vi "Main.vi"() -> ()   [LabVIEW 2019, in "Configuration.lvlib"]
uses:
  Configuration.lvlib
  Typedefs/Module References.ctl
  Typedefs/Enum_Module_Name.ctl
  Typedefs/Message.ctl
  Typedefs/Main Configuration States.ctl
  Typedefs/Configuration.ctl
  Typedefs/Application Configuration.ctl
  Module Template/Typedefs/Config.ctl
  Module Template/SubVIs/Module Template Configuraton Extractor API.vi
  Architecture.lvlib
  Module Template/Module Template.lvlib
panel:
  in  "Module_Refs":T1={"ModuleName"=enum."Controller", "Queue"=refnum, "user event"=refnum, "VI Refnum"=refnum, "ShowFP"=FALSE, "StatesTracking Enabled"=FALSE}
  out "error out":errorcluster
  in  "error in (no error)":errorcluster
  out "Message":string
  in  "Stop App":bool
  in  "Stop Module":bool
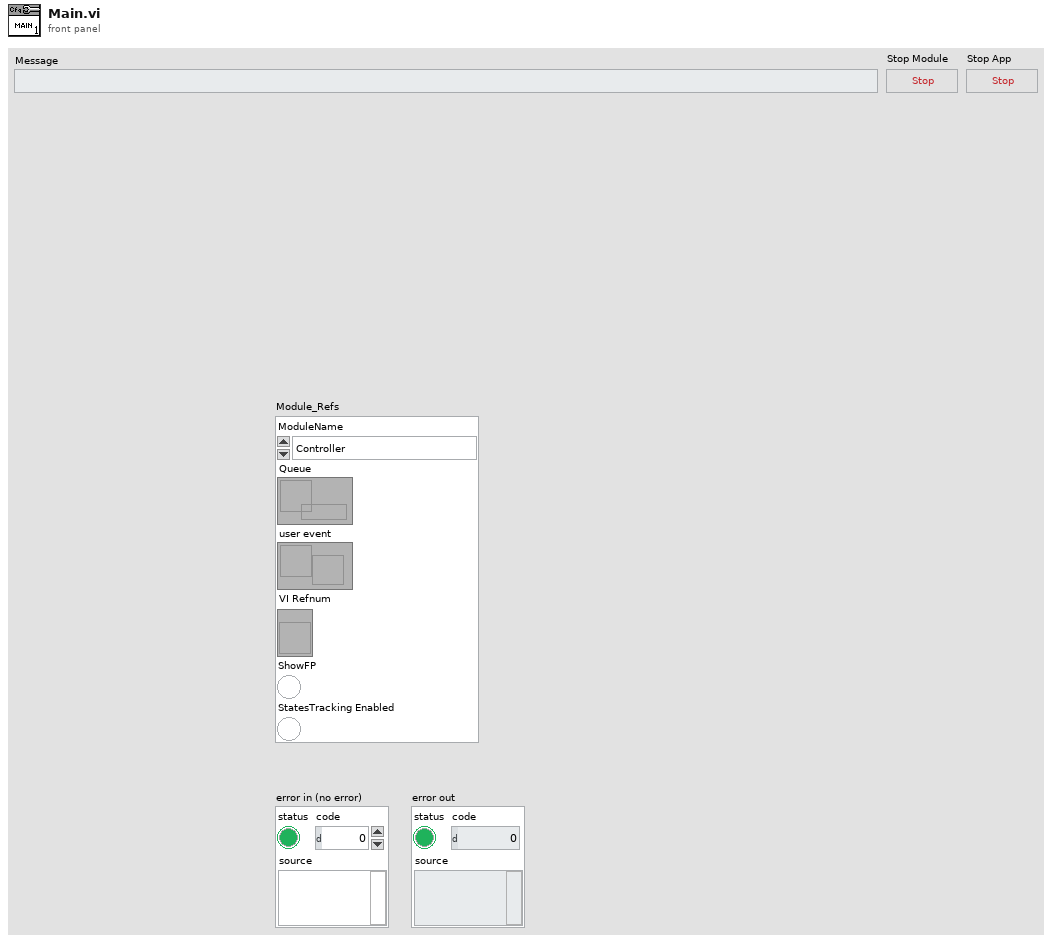
[diagram p1: front panel]
types:
  T1 = typedef "Architecture.lvlib/Module References.ctl" = cluster{"ModuleName":T2, "Queue":refnum<queue>, "user event":refnum<user-event>, "VI Refnum":refnum<vi>, "ShowFP":bool, "StatesTracking Enabled":bool}
  T2 = typedef "Architecture.lvlib/Enum_Module_Name.ctl" = enum16{"Configuration", "Error_Handler", "Log", "Database", "Controller", "User Console", "Display Console", "Sensor Interface"}
  T3 = typedef "Configuration.lvlib/Main Configuration States.ctl" = cluster{"Module_Refs":T1, "Response Data":variant, "Configuration":T4}
  T4 = typedef "Configuration.lvlib/Configuration.ctl" = cluster{"Enabled":bool}
  T5 = enum32{"Invalid", "Standard", "Closed", "Hidden", "Minimized", "Maximized"}
  T6 = typedef "Architecture.lvlib/Module Template.lvlib/Config.ctl" = cluster{"Module Enabled":bool}
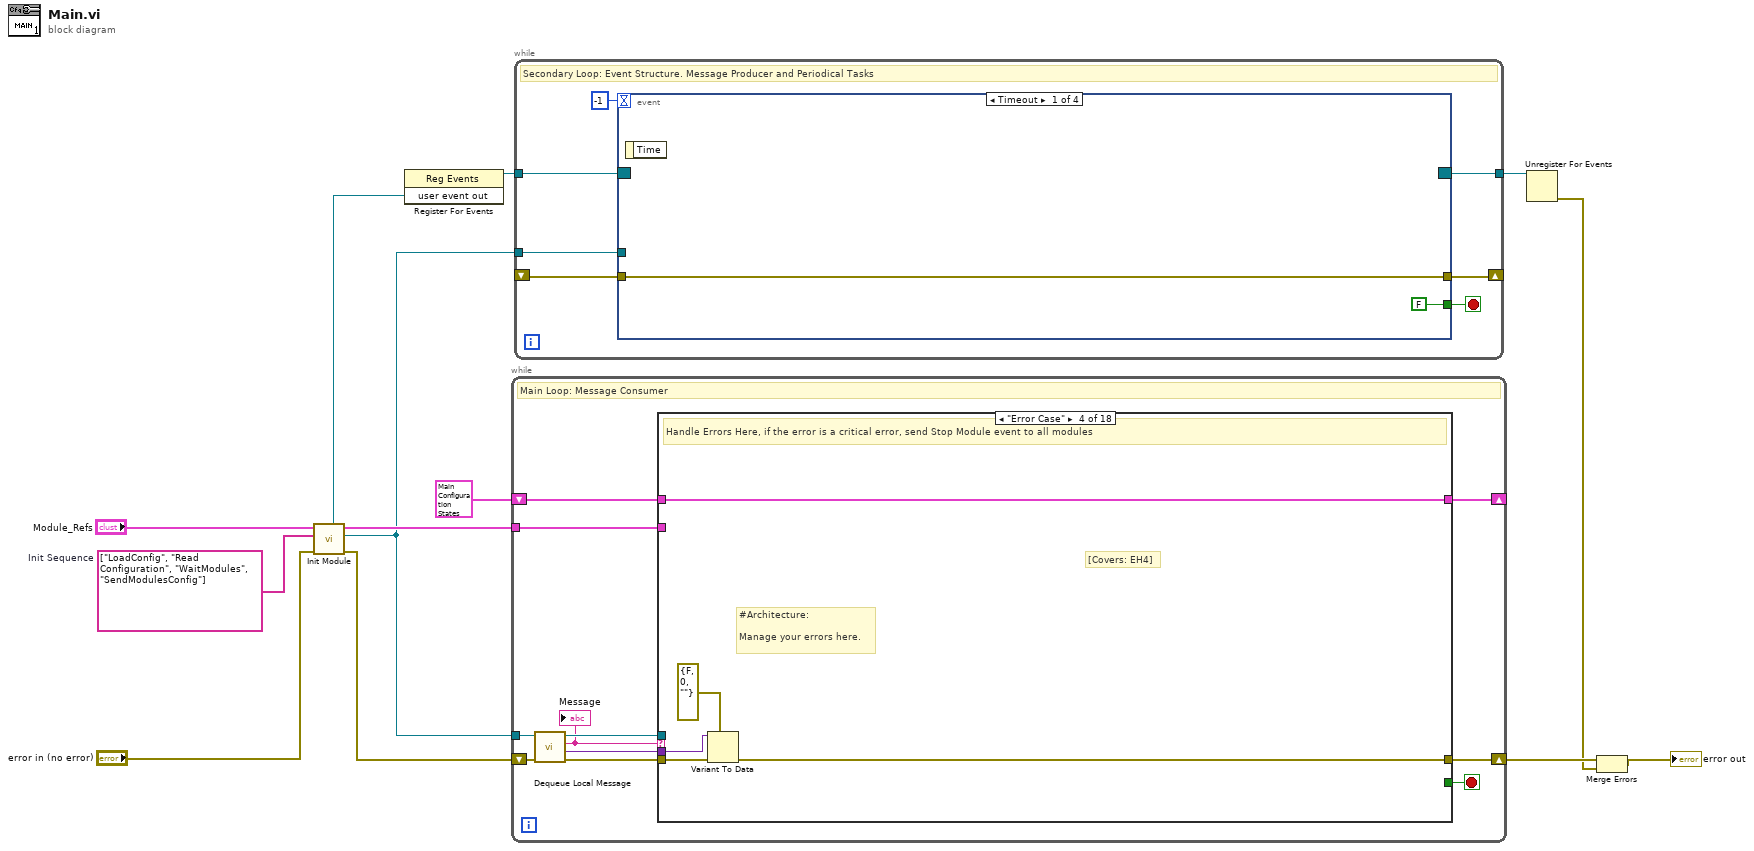
[diagram p0: block diagram]
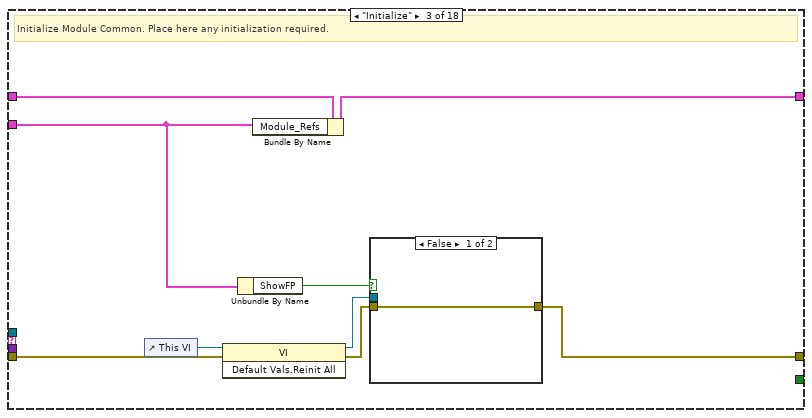
[diagram p4: hidden frame]
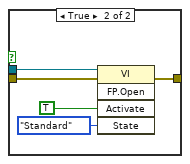
[diagram p5: hidden frame]
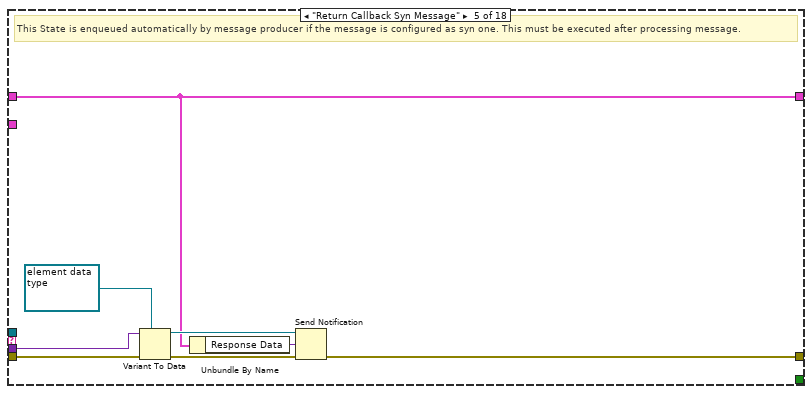
[diagram p6: hidden frame]
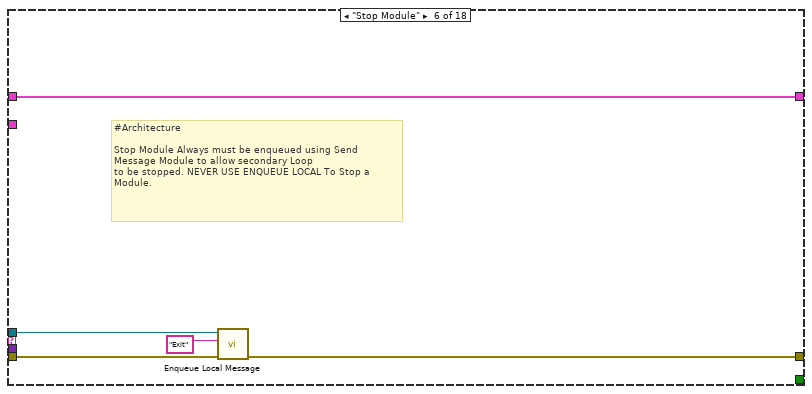
[diagram p7: hidden frame]
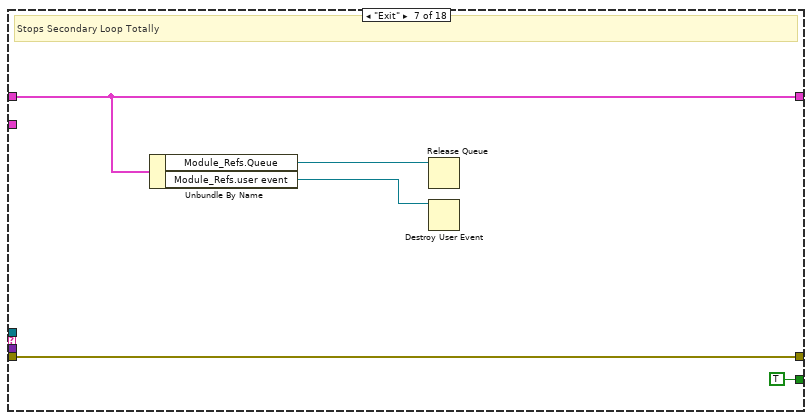
[diagram p8: hidden frame]
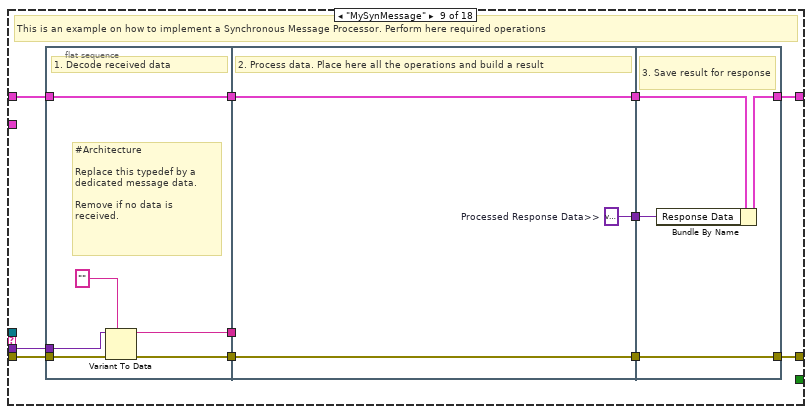
[diagram p10: hidden frame]
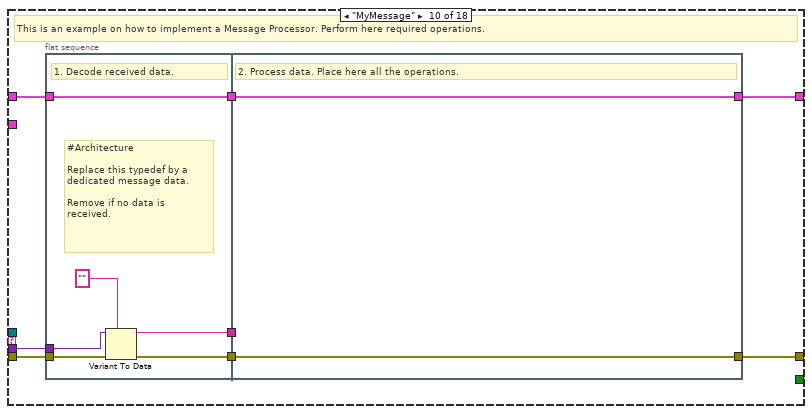
[diagram p11: hidden frame]
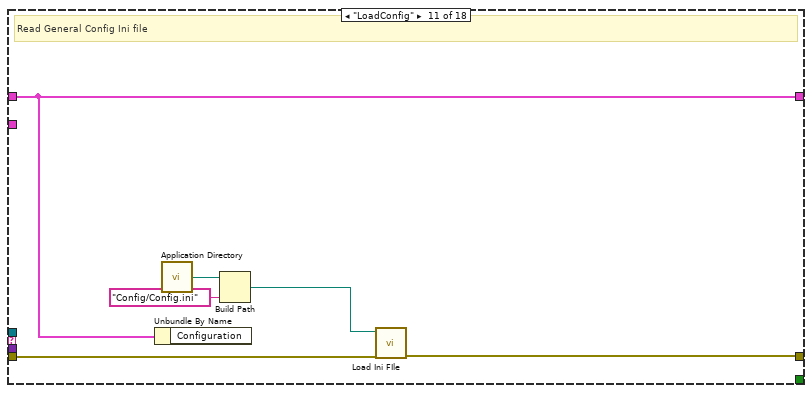
[diagram p12: hidden frame]
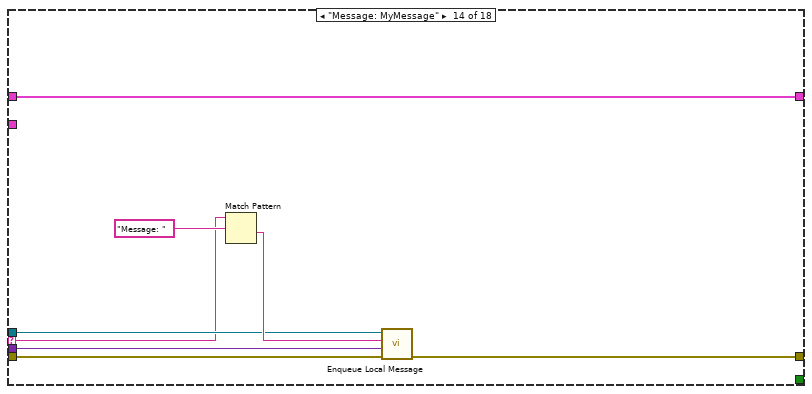
[diagram p15: hidden frame]
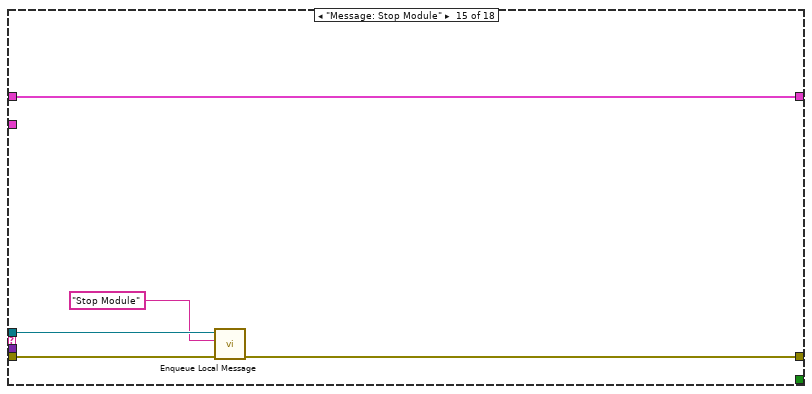
[diagram p16: hidden frame]
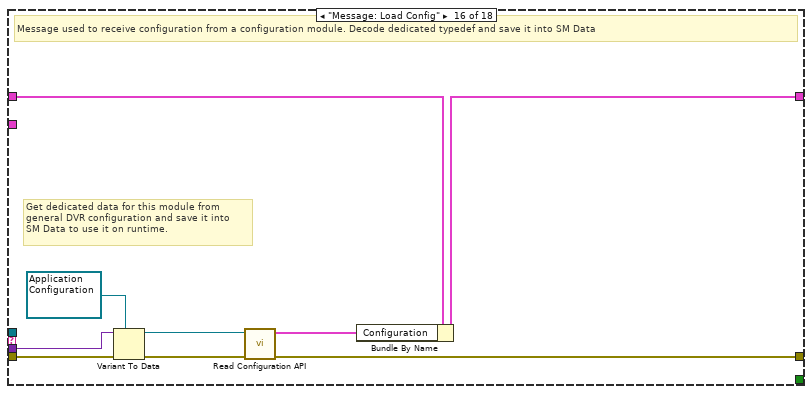
[diagram p17: hidden frame]
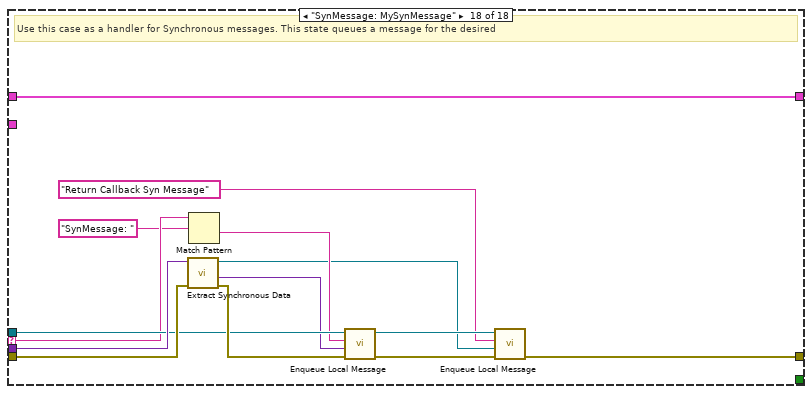
[diagram p19: hidden frame]
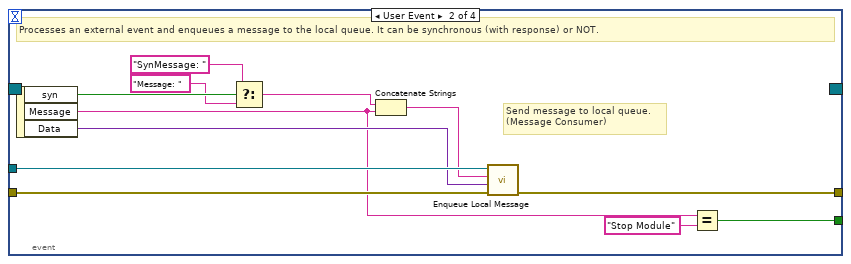
[diagram p20: hidden frame]
diagram:
  w11 = string[] ["LoadConfig", "Read Configuration", "WaitModules", "SendModulesConfig"]  # Init Sequence
  n1 = call "Init Module.vi"("error in (no error)"="error in (no error)", "Init Sequence"=w11, "Module Refs"="Module_Refs") -> ("error out"=w13:errorcluster, "queue out"=w2:refnum<queue>, "Module Refs Out"=w4:T1, "user event out"=w3:refnum<user-event>)  [unwired: 5 in]
  n2 = register-events(w3) -> (reference out=w10:refnum<event-registration>)  [unwired: 2 in, 1 out]
  n3 = while {
    shift-right: [w23] -> _
    shift-left: T3 {"Module_Refs"={"ModuleName"=enum."Controller", "Queue"=refnum, "user event"=refnum, "VI Refnum"=refnum, "ShowFP"=FALSE, "StatesTracking Enabled"=FALSE}, "Response Data"=variant, "Configuration"={"Enabled"=FALSE}} ("SM Data") -> [w24]
    shift-right: [w22] -> w8
    shift-left: w13 -> [w20]
    tunnel: w2 -> [w21]
    tunnel: w4 -> [w14]
    stop <- w15 stop-if-true
    # "Main Loop: Message Consumer"
    n4 = call "Dequeue Local Message.vi"("error in"=w20, "Msg queue in"=w21) -> ("error out"=w19:errorcluster, "Data"=w16:variant, "Message"=w17:string, "queue out"=w18:refnum<queue>)  [unwired: 6 in]
    "Message" <- w17
    n5 = case shown="\"Error Case\"" w17 {
      selector: w17 -> [_ _ _ _ _ _ _ _ _ _ _ _ _ w119 _ _ _ w151]
      tunnel: w24 -> [w26 w28 w37 w48 w50 w61 w64 w68 w79 w100 w109 w116 w118 w126 w131 w140 w142 w156]
      tunnel: [w26 w28 w35 w48 w50 w61 w64 w68 w78 w93 w109 w116 w118 w126 w131 w133 w142 w156] -> w23
      tunnel: w19 -> [w25 w27 w36 w47 w56 w60 w66 w67 w72 w96 w111 w115 w117 w123 w130 w139 w141 w155]
      tunnel: [w25 w27 w31 w46 w55 w59 w66 w67 w77 w99 w110 w115 w117 w120 w129 w134 w141 w145] -> w22
      tunnel: w18 -> [_ _ _ _ _ w58 _ _ _ _ _ _ _ w121 w128 _ _ w152]
      tunnel: w16 -> [_ _ _ w45 w53 _ _ _ w71 w95 _ _ _ w122 _ w138 _ w153]
      tunnel: [_ _ _ _ _ _ TRUE _ _ _ _ _ _ _ _ _ _ _] -> w15
      tunnel: w14 -> [_ _ w34 _ _ _ _ _ _ _ _ _ _ _ _ _ _ _]
      frame "--------State Machine Arquitechture Operations--------" {
      }
      frame "Idle", Default {
        # "Use this state to make iterations if required."
      }
      frame "Initialize" {
        # "Initialize Module Common. Place here any initialization required."
        n6 = control-ref of="This VI"() -> (w29:refnum<vi>)
        n7 = invoke class="VI" method="Default Vals.Reinit All"(reference=w29, error in=w36) -> (reference out=w32:refnum<vi>, error out=w33:errorcluster)  [unwired: 1 in, 1 out]
        n8 = Unbundle By Name(w34) -> ("ShowFP"=w30:bool)
        n9 = Bundle By Name(cluster=w37, "Module_Refs"=w34) -> (w35:T3)
        n10 = case shown="False" w30 {
          tunnel: w33 -> [w38 w43]
          tunnel: [w38 w42] -> w31
          tunnel: w32 -> [_ w41]
          frame False {
          }
          frame True {
            n11 = invoke class="VI" method="FP.Open"(reference=w41, error in=w43, "Activate"=TRUE ("Activate?"), "State"=T5."Standard") -> (error out=w42:errorcluster)  [unwired: 1 in, 4 out]
          }
        }
      }
      frame "Error Case" {
        # "[Covers: EH4]"
        # "#Architecture: \n\nManage your errors here."
        # "Handle Errors Here, if the error is a critical error, send Stop Module event to all modules"
        n12 = Variant To Data(error in=w47, type=errorcluster {"status"=FALSE, "code"=0, "source"=""} ("error constant"), Variant=w45) -> (error out=w46:errorcluster)  [unwired: 1 out]
      }
      frame "Return Callback Syn Message" {
        # "This State is enqueued automatically by message producer if the message is configured as syn one. This must be executed after processing message."
        n13 = Variant To Data(error in=w56, type=refnum<notifier> refnum ("notifier out"), Variant=w53) -> (data=w51:refnum<notifier>, error out=w54:errorcluster)
        n14 = Unbundle By Name(w50) -> ("Response Data"=w49:variant)
        n15 = Send Notification(notification=w49, notifier=w51, error in (no error)=w54) -> (error out=w55:errorcluster)  [unwired: 1 out]
      }
      frame "Stop Module" {
        # "#Architecture\n\nStop Module Always must be enqueued using Send Message Module to allow secondary Loop\nto be stopped. NEVER USE ENQUEUE LOCAL To Stop a Module."
        n16 = call "Enqueue Local Message.vi"("error in"=w60, "Message"="Exit", "Msg queue in"=w58) -> ("error out"=w59:errorcluster)  [unwired: 7 in, 1 out]
      }
      frame "Exit" {
        # "Stops Secondary Loop Totally"
        n17 = Unbundle By Name(w64) -> ("Module_Refs.Queue"=w63:refnum<queue>, "Module_Refs.user event"=w62:refnum<user-event>)
        n18 = Release Queue(queue=w63) -> ()  [unwired: 2 in, 3 out]
        n19 = Destroy User Event(user event=w62) -> ()  [unwired: 1 in, 1 out]
      }
      frame "--------------State Machine Custom States-------------" {
      }
      frame "MySynMessage" {
        # "This is an example on how to implement a Synchronous Message Processor. Perform here required operations"
        n20 = flat-sequence {
          tunnel: w72 -> [w83]
          tunnel: w79 -> [w85]
          tunnel: [w85] -> w76
          tunnel: [w81] -> w75
          tunnel: w71 -> [w82]
          tunnel: [w80] -> w70
          tunnel: w76 -> [w88]
          tunnel: w75 -> [w87]
          tunnel: [w88] -> w74
          tunnel: [w87] -> w73
          tunnel: w70 -> [_]
          tunnel: [w86] -> w69
          tunnel: [w91] -> w77
          tunnel: [w90] -> w78
          tunnel: w74 -> [w92]
          tunnel: w73 -> [w91]
          tunnel: w69 -> [w89]
          frame #0 {
            # "#Architecture\n\nReplace this typedef by a dedicated message data.\n\nRemove if no data is received."
            # "1. Decode received data"
            n21 = Variant To Data(error in=w83, type="", Variant=w82) -> (data=w80:string, error out=w81:errorcluster)
          }
          frame #1 {
            w86 = variant  # Processed Response Data>>
            # "2. Process data. Place here all the operations and build a result"
          }
          frame #2 {
            # "3. Save result for response"
            n22 = Bundle By Name(cluster=w92, "Response Data"=w89) -> (w90:T3)
          }
        }
      }
      frame "MyMessage" {
        # "This is an example on how to implement a Message Processor. Perform here required operations."
        n23 = flat-sequence {
          tunnel: w96 -> [w104]
          tunnel: w100 -> [w106]
          tunnel: [w106] -> w98
          tunnel: [w102] -> w97
          tunnel: w95 -> [w103]
          tunnel: [w101] -> w94
          tunnel: w98 -> [w107]
          tunnel: w97 -> [w108]
          tunnel: w94 -> [_]
          tunnel: [w108] -> w99
          tunnel: [w107] -> w93
          frame #0 {
            # "#Architecture\n\nReplace this typedef by a dedicated message data.\n\nRemove if no data is received."
            # "1. Decode received data."
            n24 = Variant To Data(error in=w104, type="", Variant=w103) -> (data=w101:string, error out=w102:errorcluster)
          }
          frame #1 {
            # "2. Process data. Place here all the operations."
          }
        }
      }
      frame "LoadConfig" {
        # "Read General Config Ini file"
        n25 = Unbundle By Name(w109) -> ()  [unwired: 1 out]
        n26 = call <vilib>:"Application Directory.vi"() -> ("Application Directory"=w114:path)
        n27 = Build Path(base path=w114, name or relative path="Config/Config.ini") -> (appended path=w112:path)
        n28 = call "Load Ini FIle.vi"("error in (no error)"=w111, "configuration file path"=w112) -> ("error out"=w110:errorcluster)  [unwired: 8 in, 1 out]
      }
      frame "Read Configuration" {
      }
      frame "--------------Dynamic Events Messages----------------" {
      }
      frame "Message: MyMessage" {
        n29 = Match Pattern(string=w119, regular expression="Message: ") -> (after substring=w124:string)  [unwired: 1 in, 3 out]
        n30 = call "Enqueue Local Message.vi"("error in"=w123, "Data"=w122, "Message"=w124, "Msg queue in"=w121) -> ("error out"=w120:errorcluster)  [unwired: 6 in, 1 out]
      }
      frame "Message: Stop Module" {
        n31 = call "Enqueue Local Message.vi"("error in"=w130, "Message"="Stop Module", "Msg queue in"=w128) -> ("error out"=w129:errorcluster)  [unwired: 7 in, 1 out]
      }
      frame "Message: Load Config" {
        # "Get dedicated data for this module from \ngeneral DVR configuration and save it into \nSM Data to use it on runtime."
        # "Message used to receive configuration from a configuration module. Decode dedicated typedef and save it into SM Data"
        n32 = Variant To Data(error in=w139, type=refnum<data-value> refnum ("data value reference"), Variant=w138) -> (data=w136:refnum<data-value>, error out=w135:errorcluster)
        n33 = call-poly "Read Configuration API.vi"("error constant"=w135, "General Config DVR In"=w136) -> ("error out"=w134:errorcluster, "Module Template Config"=w132:T6)  [unwired: 8 in]
        n34 = Bundle By Name(cluster=w140, "Configuration"=w132) -> (w133:T3)
      }
      frame "------------Synchronous Event Messages--------------" {
      }
      frame "SynMessage: MySynMessage" {
        # "Use this case as a handler for Synchronous messages. This state queues a message for the desired"
        n35 = call "Extract Synchronous Data.vi"("error in 2"=w155, "Variant"=w153) -> ("error in"=w154:errorcluster, "Data Out"=w148:variant, "notifier out"=w143:refnum<notifier>)  [unwired: 7 in]
        n36 = Match Pattern(string=w151, regular expression="SynMessage: ") -> (after substring=w149:string)  [unwired: 1 in, 3 out]
        n37 = call "Enqueue Local Message.vi"("error in"=w154, "Data"=w148, "Message"=w149, "Msg queue in"=w152) -> ("error out"=w147:errorcluster, "queue out"=w146:refnum<queue>)  [unwired: 6 in]
        n38 = call "Enqueue Local Message.vi"("error in"=w147, "Data"=w143, "Message"="Return Callback Syn Message", "Msg queue in"=w146) -> ("error out"=w145:errorcluster)  [unwired: 6 in, 1 out]
      }
    }
  }
  n39 = while {
    tunnel: w10 -> [w163]
    tunnel: w2 -> [w160]
    tunnel: [w159] -> w9
    shift-right: [w157] -> _
    shift-left: _ -> [w158]
    stop <- w161 stop-if-true
    # "Secondary Loop: Event Structure. Message Producer and Periodical Tasks"
    n40 = event shown="[0] Timeout" {
      selector: w163 -> [_ _ _ _]
      dyn-events: [_ _ _ _] -> w159
      timeout: -1 -> [_ _ _ _]
      tunnel: [FALSE w172 TRUE _] -> w161
      tunnel: w160 -> [_ w177 w179 _]
      tunnel: w158 -> [w164 w176 w182 w184]
      tunnel: [w164 w175 w180 w183] -> w157
      event Timeout {
        n41 = event-data() -> ()  [unwired: 1 in, 1 out]
      }
      event User Event {
        # "Send message to local queue. \n(Message Consumer)"
        # "Processes an external event and enqueues a message to the local queue. It can be synchronous (with response) or NOT."
        n42 = event-data() -> ("syn"=w169:bool, "Message"=w171:string, "Data"=w174:variant)  [unwired: 1 in]
        n43 = Select(t="SynMessage: " ("string"), s=w169, f="Message: " ("string")) -> (s? t:f=w166:string)
        n44 = Concatenate Strings(w166, w171) -> (w173:string)
        n45 = call "Enqueue Local Message.vi"("error in"=w176, "Data"=w174, "Message"=w173, "Msg queue in"=w177) -> ("error out"=w175:errorcluster)  [unwired: 6 in, 1 out]
        n46 = Equal?(x=w171, y="Stop Module") -> (x = y?=w172:bool)
      }
      event "Stop Module": Value Change {
        n47 = event-data() -> ()  [unwired: 1 in, 1 out]
        n48 = call "Enqueue Local Message.vi"("error in"=w182, "Message"="Stop Module", "Msg queue in"=w179) -> ("error out"=w180:errorcluster)  [unwired: 7 in, 1 out]
      }
      event "Stop App": Value Change {
        w186 = TRUE  # All Modules
        # "Send Stop To All Modules"
        n49 = event-data() -> ()  [unwired: 1 in, 1 out]
        n50 = call "Send Message Modules.vi"("All Modules"=w186, "Error In"=w184, "Message"="Stop Module") -> ("error in (no error)"=w183:errorcluster)  [unwired: 8 in]
      }
    }
  }
  n51 = Unregister For Events(event registration refnum=w9) -> (error out=w7:errorcluster)  [unwired: 1 in]
  n52 = Merge Errors(w8, w7) -> (→"error out":errorcluster)
